vi "FlatToRichGreeter_res.vi"(5 "OutputClusterType":T1, 11 "InputCluster":T3) -> (3 "OutputCluster":T1)   [LabVIEW 2019, in "Generated_server.lvlib"]
uses:
  Generated_server.lvlib
  Greeter_res_Flat.ctl
  Greeter_MessageA_Flat.ctl
  Greeter_res.ctl
  Greeter_res_res_oneof/Greeter_res_res_oneof.lvclass
  Greeter_MessageA.ctl
  Greeter_res_res_oneof/Greeter_res_res_oneof.lvclass/Greeter_res_res_oneof.ctl
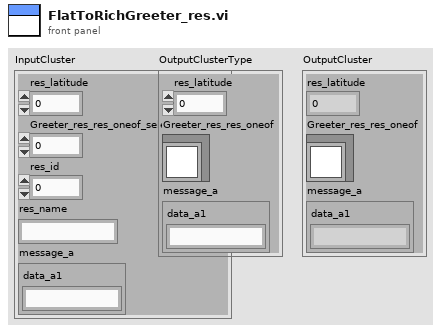
[diagram p1: front panel]
types:
  T1 = typedef "Generated_server.lvlib/Greeter_res.ctl" = cluster{"res_latitude":i32, "Greeter_res_res_oneof":refnum<class "Greeter_res_res_oneof.lvclass">, "message_a":T2}
  T2 = typedef "Generated_server.lvlib/Greeter_MessageA.ctl" = cluster{"data_a1":string}
  T3 = typedef "Generated_server.lvlib/Greeter_res_Flat.ctl" = cluster{"res_latitude":i32, "Greeter_res_res_oneof_selected_index":i32, "res_id":i32, "res_name":string, "message_a":T4}
  T4 = typedef "Generated_server.lvlib/Greeter_MessageA_Flat.ctl" = cluster{"data_a1":string}
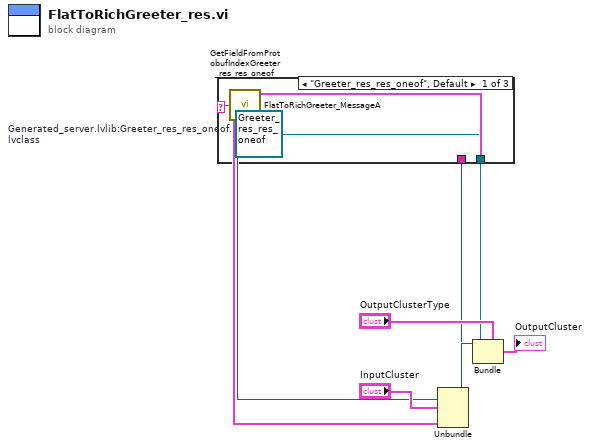
[diagram p0: block diagram]
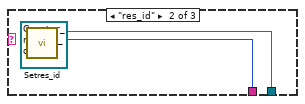
[diagram p2: hidden frame]
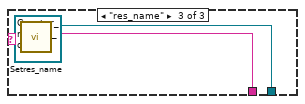
[diagram p3: hidden frame]
diagram:
  n1 = Unbundle "Unbundle"("InputCluster") -> ("res_latitude"=w8:i32, "Greeter_res_res_oneof_selected_index"=w7:i32, "res_id"=w4:i32, "res_name"=w3:string, "message_a"=w2:T4)
  n2 = call "FlatToRichGreeter_MessageA.vi"("InputCluster"=w2) -> ("OutputCluster"=w1:T2)  [unwired: 10 in]
  n3 = call "GetFieldFromProtobufIndexGreeter_res_res_oneof.vi"("protobuf index"=w7) -> ("oneof field name"=w6:string)
  n4 = case "Greeter_res_res_oneof" shown="\"Greeter_res_res_oneof\", Default" w6 {
    tunnel: [w12 w14 w17] -> w5
    tunnel: w4 -> [_ w15 _]
    tunnel: w3 -> [_ _ w18]
    frame "Greeter_res_res_oneof", Default {
      w12 = refnum<class "Greeter_res_res_oneof.lvclass"> refnum  # Generated_server.lvlib:Greeter_res_res_oneof.lvclass
    }
    frame "res_id" {
      n5 = call "Setres_id.vi"("Set_Val"=w15, "OneOfTemplate in"=refnum<class "Greeter_res_res_oneof.lvclass"> refnum) -> ("OneOfTemplate out"=w14:refnum<class "Greeter_res_res_oneof.lvclass">)  [unwired: 8 in, 1 out]
    }
    frame "res_name" {
      n6 = call "Setres_name.vi"("Set_Val"=w18, "OneOfTemplate in"=refnum<class "Greeter_res_res_oneof.lvclass"> refnum) -> ("OneOfTemplate out"=w17:refnum<class "Greeter_res_res_oneof.lvclass">)  [unwired: 8 in, 1 out]
    }
  }
  n7 = Bundle "Bundle"(cluster="OutputClusterType", "res_latitude"=w8, "Greeter_res_res_oneof"=w5, "message_a"=w1) -> (→"OutputCluster":T1)
